vi "Write A.vi"(8 "error in (no error)":errorcluster, 10 "A":dbl, 11 "Multiply in":refnum<class "Multiply.lvclass">) -> (0 "error out":errorcluster, 3 "Multiply out":refnum<class "Multiply.lvclass">)   [LabVIEW 2023, in "Multiply.lvclass"]
uses:
  Multiply.lvclass
  Multiply.lvclass/Multiply.ctl
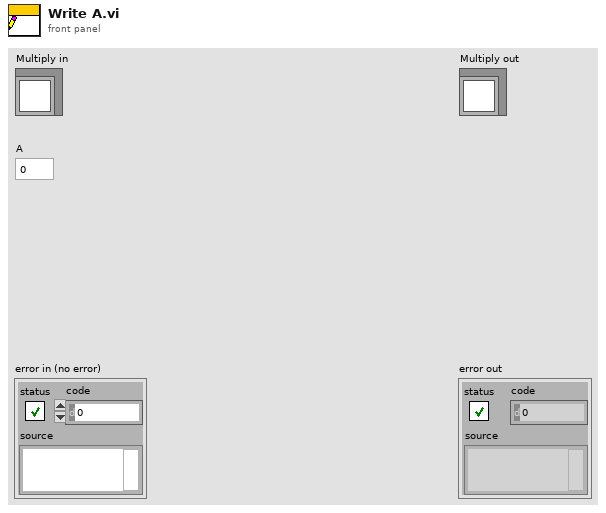
[diagram p1: front panel]
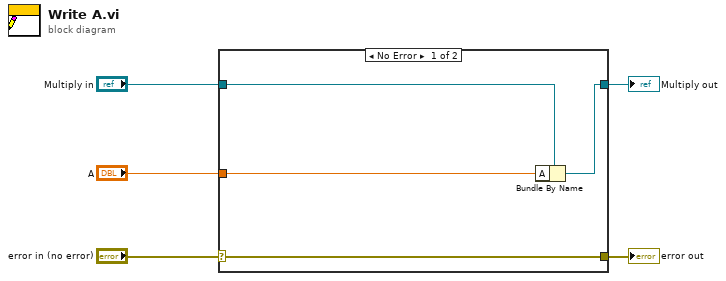
[diagram p0: block diagram]
diagram:
  n1 = case shown="No Error" "error in (no error)" {
    selector: "error in (no error)" -> [w9 w10]
    tunnel: [w9 w10] -> w4
    tunnel: [w7 w11] -> w2
    tunnel: "Multiply in" -> [w8 w11]
    tunnel: "A" -> [w6 _]
    frame No Error {
      n2 = Bundle By Name(cluster=w8, "A"=w6) -> (w7:refnum<class "Multiply.lvclass">)
    }
    frame Error {
    }
  }
  "error out" <- w4
  "Multiply out" <- w2
